vi "Prog2.vi"() -> ()   [LabVIEW 2021]
panel:
  out "length 3":i32
  out "decimal integer string":string
  out "length 2":i32
  out "reversed":string
  out "length":i32
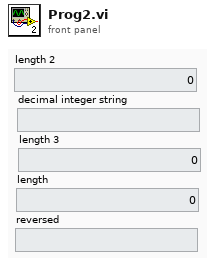
[diagram p1: front panel]
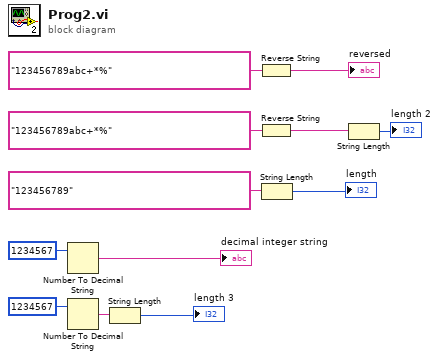
[diagram p0: block diagram]
diagram:
  n1 = Number To Decimal String(number=1234567) -> (decimal integer string=→"decimal integer string":string)  [unwired: 1 in]
  n2 = Number To Decimal String(number=1234567) -> (decimal integer string=w1:string)  [unwired: 1 in]
  n3 = String Length(string=w1) -> (length=→"length 3":i32)
  n4 = Reverse String(1:"123456789abc+*%") -> (0:→"reversed":string)
  n5 = Reverse String(1:"123456789abc+*%") -> (0:w6:string)
  n6 = String Length(string="123456789") -> (length=→"length":i32)
  n7 = String Length(string=w6) -> (length=→"length 2":i32)
